vi "Distance.vi"(8 "Pose 2":T1, 11 "Pose 1":T1) -> (3 "Distance":dbl)   [LabVIEW 2013]
uses:
  <vilib>/Analysis/Matrix/Datatypes/RealMatrix.ctl
  <vilib>/Analysis/Matrix/NI_Matrix.lvlib
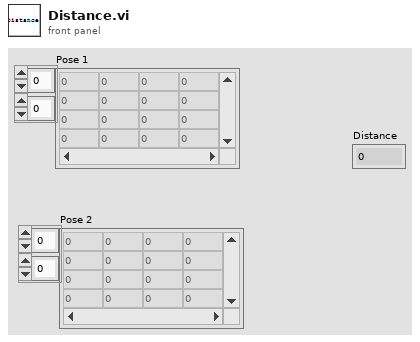
[diagram p1: front panel]
types:
  T1 = typedef "NI_Matrix.lvlib/RealMatrix.ctl" = dbl[][]
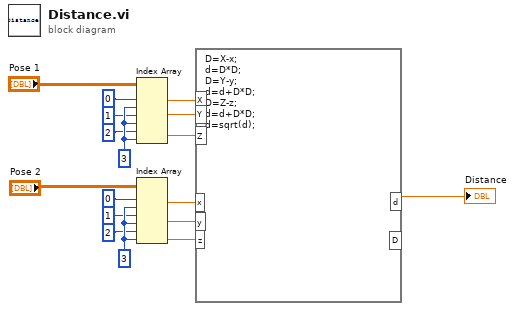
[diagram p0: block diagram]
diagram:
  w12 = 3 ("index (col)")
  w16 = 3 ("index (col)")
  n1 = Index Array(array="Pose 1", index (row) #1=0 ("index (row)"), index (col) #1=w16, index (row) #2=1 ("index (row)"), index (col) #2=w16, index (row) #3=2 ("index (row)"), index (col) #3=w16) -> (element #1=w7:dbl, element #2=w6:dbl, element #3=w5:dbl)
  n2 = Index Array(array="Pose 2", index (row) #1=0 ("index (row)"), index (col) #1=w12, index (row) #2=1 ("index (row)"), index (col) #2=w12, index (row) #3=2 ("index (row)"), index (col) #3=w12) -> (element #1=w4:dbl, element #2=w3:dbl, element #3=w2:dbl)
  n3 = formula code="D=X-x;\nd=D*D;\nD=Y-y;\nd=d+D*D;\nD=Z-z;\nd=d+D*D;\nd=sqrt(d);"("X"=w7, "Y"=w6, "Z"=w5, "x"=w4, "y"=w3, "z"=w2) -> ("d"=→"Distance":dbl)  [unwired: 1 out]
